vi "Constructor.vi"(8 "error in (no error)":errorcluster, 11 "MarkovModel in":refnum<class "MarkovModel.lvclass">) -> (0 "error out":errorcluster, 3 "MarkovModel out":refnum<class "MarkovModel.lvclass">)   [LabVIEW 2020, in "MarkovModel.lvclass"]
uses:
  MarkovModel.lvclass
  MarkovModel.lvclass/MarkovModel.ctl
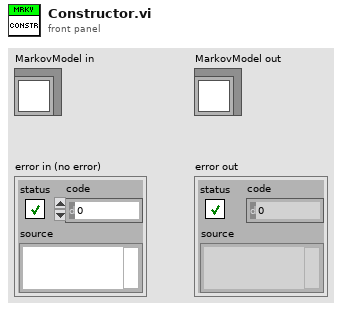
[diagram p1: front panel]
types:
  T1 = map{string[], cluster{"Class Name":string, "Count":i32}[]}
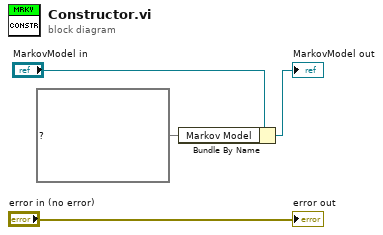
[diagram p0: block diagram]
diagram:
  n1 = Bundle By Name(cluster="MarkovModel in", "Markov Model"=T1 {}) -> (→"MarkovModel out":refnum<class "MarkovModel.lvclass">)
  "error out" <- "error in (no error)"
